vi "ke37xx Resistor Sort Example.vi"() -> ()   [LabVIEW 2009]
doc: "ResistorSort Source Code \n\nThis sample uses the DMM limit testing functionality to test\nresistors and sort them into three different bins, based upon\ntheir value relative to a nominal resistance value.\nResistors that are measured within 1% of nominal are sorted\ninto Bin 1. Resistors with a 1% to 5% deviation from the nominal\nresistance are sorted into Bin 2. Resistors that are 5% beyond\nNominal are sorted into Bin3.\n\nDigital I/O lines 1 to 4 are used to report limit failures to an\nexternal device, such as a component handler for performing\nbinning operations. The digitial I/O lines are programmed\nto respond as follows. (The symbol R0 denotes the nominal\nresistance value.)\n\nResistance Deviation: DIO Output Lines Driven:\n\n < 1% (none)\n - 1% Line 1\n + 1% Line 2\n - 5% Line 1 and Line 3\n + 5% Line 2 and Line 4\n\nThe results of the binning operation are presented in separate\narray controls on the front panel. Run the VI repeatedly to make\nmultiple measurements and have them accumulate in the\nappropriate bins."
uses:
  <instrlib>/Keithley 3706/Keithley 3700 Series.lvlib
panel:
  out "Bin 3: > 5% tolerance":dbl[](array[numeric]) format="%#_6e"
  out "Bin 2: 1 % to 5% tolerance":dbl[](array[numeric]) format="%#_6e"
  in  "Nominal Value (100 Ohms)":dbl=100.0
  out "Bin 1: < 1 % tolerance":dbl[](array[numeric]) format="%#_6e"
  in  "VISA Resource Name":refnum<visa-resource-name>="GPIB::6"
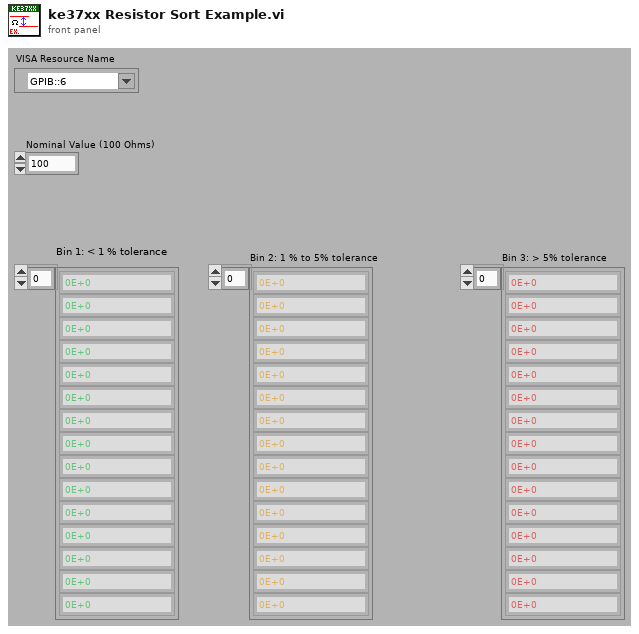
[diagram p1: front panel]
types:
  T1 = enum16{"None", "All", "2-Wire", "4-Wire", "2-Wire Amps", "Amps"}
  T2 = enum16{"None", "DC Volts", "AC Volts", "DC Current", "AC Current", "2-Wire Ohms", "4-Wire Ohms", "Temperature", "Period", "Frequency", "Continuity", "Commonside Ohms"}
  T3 = enum16{"None", "Alarm 1", "Alarm 2", "Digital I/O Line 1", "Digital I/O Line 2", "Digital I/O Line 3", "Digital I/O Line 4", "Digital I/O Line 5", "Digital I/O Line 6", "Digital I/O Line 7", "Digital I/O Line 8", "Digital I/O Line 9", "Digital I/O Line 10", "Digital I/O Line 11", "Digital I/O Line 12", "Digital I/O Line 13", "Digital I/O Line 14", "TSP Link Line 1", "TSP Link Line 2", "TSP Link Line 3", "Blender 1", "Blender 2", "Timer 1", "Timer 2", "Timer 3", "Timer 4", "LAN Line 1", "LAN Line 2", "LAN Line 3", "LAN Line 4", "LAN Line 5", "LAN Line 6", "LAN Line 7", "LAN Line 8", "DMM Limit 1 High", "DMM Limit 1 Low", "DMM Limit 2 High", "DMM Limit 2 Low", "Display", "Measure Complete", "Sequence Complete", "Scan Ready", "Scan Start", "Scan Complete", "Channel Ready", "Idle", "Software"}
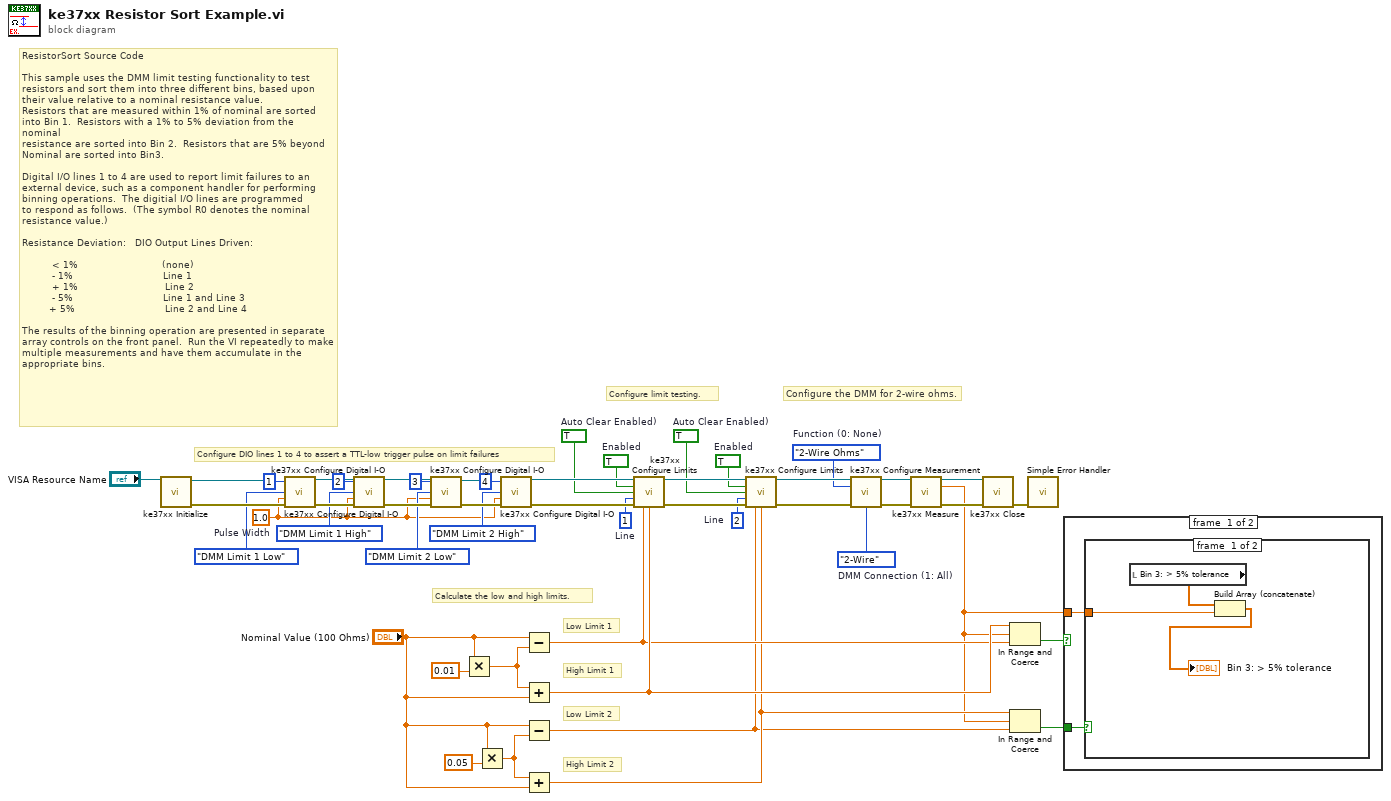
[diagram p0: block diagram]
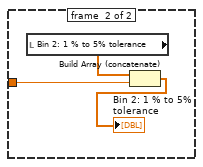
[diagram p2: hidden frame]
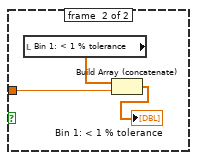
[diagram p3: hidden frame]
diagram:
  w11 = T1."2-Wire"  # DMM Connection (1: All)
  w12 = T2."2-Wire Ohms"  # Function (0: None)
  w13 = 1.0  # Pulse Width
  w16 = TRUE  # Auto Clear Enabled)
  w15 = u8 2  # Line
  w14 = TRUE  # Enabled
  w17 = TRUE  # Auto Clear Enabled)
  w18 = u8 1  # Line
  w19 = TRUE  # Enabled
  # "Configure the DMM for 2-wire ohms."
  # "Configure limit testing."
  # "Calculate the low and high limits."
  # "Configure DIO lines 1 to 4 to assert a TTL-low trigger pulse on limit failures"
  # "High Limit 2"
  # "Low Limit 2"
  # "High Limit 1"
  # "Low Limit 1"
  # "ResistorSort Source Code                                 \n\nThis sample uses the DMM limit testing functionality to test\nresistors and sort them into three different bins, based upon\ntheir value relative to a nominal resistance value.\nResistors that are measured within 1% of nominal are sorted\ninto Bin 1.  Resistors with a 1% to 5% deviation from the nominal\nresistance are sorted into Bin 2.  Resistors that are 5% beyond\nNominal are sorted into Bin3.\n\nDigital I/O lines 1 to 4 are used to report limit failures to an\nexternal device, such as a component handler for performing\nbinning operations.  The digitial I/O lines are programmed\nto respond as follows.  (The symbol R0 denotes the nominal\nresistance value.)\n\nResistance Deviation:\t\t\tDIO Output Lines Driven:\n\n          < 1%\t\t\t\t\t\t                      (none)\n          - 1%\t\t\t\t\t\t                        Line 1\n          + 1%\t\t\t\t\t\t                       Line 2\n          - 5%\t\t\t\t\t\t                        Line 1 and Line 3\n         + 5%\t\t\t\t\t\t                        Line 2 and Line 4\n\nThe results of the binning operation are presented in separate\narray controls on the front panel.  Run the VI repeatedly to make\nmultiple measurements and have them accumulate in the\nappropriate bins."
  n1 = call <instrlib>:"ke37xx Initialize.vi"("VISA resource name"="VISA Resource Name") -> ("VISA resource name out"=w10:refnum<visa-resource-name>, "error out"=w47:errorcluster)  [unwired: 13 in]
  n2 = call <instrlib>:"ke37xx Configure Digital I-O.vi"("VISA Resource Name"=w10, "Line (1)"=u8 1, "Stimulus (0: None)"=T3."DMM Limit 1 Low", "Pulse Width (10 sec)"=w13, "error in (no error)"=w47) -> ("VISA Resource Name Out"=w30:refnum<visa-resource-name>, "error out"=w27:errorcluster)  [unwired: 9 in]
  n3 = call <instrlib>:"ke37xx Configure Digital I-O.vi"("VISA Resource Name"=w30, "Line (1)"=u8 2, "Stimulus (0: None)"=T3."DMM Limit 1 High", "Pulse Width (10 sec)"=w13, "error in (no error)"=w27) -> ("VISA Resource Name Out"=w29:refnum<visa-resource-name>, "error out"=w26:errorcluster)  [unwired: 9 in]
  n4 = call <instrlib>:"ke37xx Configure Digital I-O.vi"("VISA Resource Name"=w29, "Line (1)"=u8 3, "Stimulus (0: None)"=T3."DMM Limit 2 Low", "Pulse Width (10 sec)"=w13, "error in (no error)"=w26) -> ("VISA Resource Name Out"=w28:refnum<visa-resource-name>, "error out"=w25:errorcluster)  [unwired: 9 in]
  n5 = Multiply(x="Nominal Value (100 Ohms)", y=0.01) -> (x*y=w37:dbl)
  n6 = Multiply(x="Nominal Value (100 Ohms)", y=0.05) -> (x*y=w38:dbl)
  n7 = call <instrlib>:"ke37xx Configure Digital I-O.vi"("VISA Resource Name"=w28, "Line (1)"=u8 4, "Stimulus (0: None)"=T3."DMM Limit 2 High", "Pulse Width (10 sec)"=w13, "error in (no error)"=w25) -> ("VISA Resource Name Out"=w21:refnum<visa-resource-name>, "error out"=w20:errorcluster)  [unwired: 9 in]
  n8 = Subtract(x="Nominal Value (100 Ohms)", y=w37) -> (x-y=w6:dbl)
  n9 = Add(x=w37, y="Nominal Value (100 Ohms)") -> (x+y=w7:dbl)
  n10 = Subtract(x="Nominal Value (100 Ohms)", y=w38) -> (x-y=w3:dbl)
  n11 = Add(x=w38, y="Nominal Value (100 Ohms)") -> (x+y=w4:dbl)
  n12 = call <instrlib>:"ke37xx Configure Limits.vi"("VISA Resource Name"=w21, "Limit Enabled (False)"=w19, "Auto Clear Enabled (False)"=w17, "Limit Line (1)"=w18, "error in (no error)"=w20, "Lower Limit (NaN: Don't Set)"=w6, "Upper Limit (NaN: Don't Set)"=w7) -> ("VISA Resource Name Out"=w44:refnum<visa-resource-name>, "error out"=w43:errorcluster)  [unwired: 7 in]
  n13 = call <instrlib>:"ke37xx Configure Limits.vi"("VISA Resource Name"=w44, "Limit Enabled (False)"=w14, "Auto Clear Enabled (False)"=w16, "Limit Line (1)"=w15, "error in (no error)"=w43, "Lower Limit (NaN: Don't Set)"=w3, "Upper Limit (NaN: Don't Set)"=w4) -> ("VISA Resource Name Out"=w46:refnum<visa-resource-name>, "error out"=w45:errorcluster)  [unwired: 7 in]
  n14 = call <instrlib>:"ke37xx Configure Measurement.vi"("VISA Resource Name"=w46, "Function (0: None)"=w12, "error in (no error)"=w45, "DMM Connection (1: All)"=w11) -> ("VISA Resource Name Out"=w9:refnum<visa-resource-name>, "error out"=w8:errorcluster)  [unwired: 10 in]
  n15 = call <instrlib>:"ke37xx Measure.vi"("VISA Resource Name"=w9, "error in (no error)"=w8) -> ("VISA Resource Name Out"=w48:refnum<visa-resource-name>, "Reading"=w2:dbl, "error out"=w49:errorcluster)  [unwired: 9 in, 2 out]
  n16 = call <instrlib>:"ke37xx Close.vi"("VISA resource name"=w48, "error in (no error)"=w49) -> ("error out"=w41:errorcluster)  [unwired: 13 in]
  n17 = In Range and Coerce(upper limit=w7, x=w2, lower limit=w6) -> (In Range?=w5:bool)  [unwired: 1 out]
  n18 = In Range and Coerce(upper limit=w4, x=w2, lower limit=w3) -> (In Range?=w1:bool)  [unwired: 1 out]
  n19 = call <vilib>:"Simple Error Handler.vi"("error in (no error)"=w41) -> ()  [unwired: 1 in, 8 out]
  n20 = case shown="False" w5 {
    tunnel: w2 -> [w50 w59]
    tunnel: w1 -> [w51 _]
    frame #0 {
      n21 = case shown="False" w51 {
        tunnel: w50 -> [w53 w56]
        frame #0 {
          n22 = local read "Bin 3: > 5% tolerance"() -> (w54:dbl[])
          n23 = Build Array (concatenate)(w54, w53) -> (→"Bin 3: > 5% tolerance":dbl[])
        }
        frame #1 {
          n24 = local read "Bin 2: 1 % to 5% tolerance"() -> (w57:dbl[])
          n25 = Build Array (concatenate)(w57, w56) -> (→"Bin 2: 1 % to 5% tolerance":dbl[])
        }
      }
    }
    frame #1 {
      n26 = local read "Bin 1: < 1 % tolerance"() -> (w60:dbl[])
      n27 = Build Array (concatenate)(w60, w59) -> (→"Bin 1: < 1 % tolerance":dbl[])
    }
  }
